vi "Destroy User Events.vi"(11 "CANopen Test UI in":refnum<class "CANopen Test UI Actor.lvclass">) -> (3 "CANopen Test UI out":refnum<class "CANopen Test UI Actor.lvclass">)   [LabVIEW 2024, in "CANopen Test UI Actor.lvlib" / "CANopen Test UI Actor.lvclass"]
uses:
  CANopen Test UI Actor.lvclass
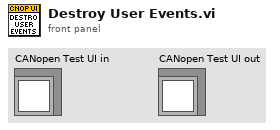
[diagram p1: front panel]
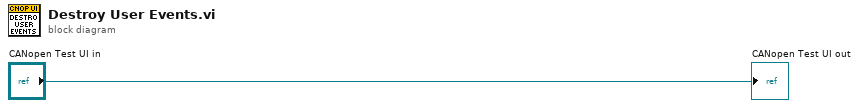
[diagram p0: block diagram]
diagram:
  "CANopen Test UI out" <- "CANopen Test UI in"
